vi "Emergency_Stop_JT.vi"(8 "error in":errorcluster, 11 "connection ID":refnum<k5>) -> ()   [LabVIEW 2018]
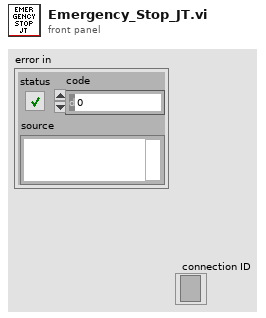
[diagram p1: front panel]
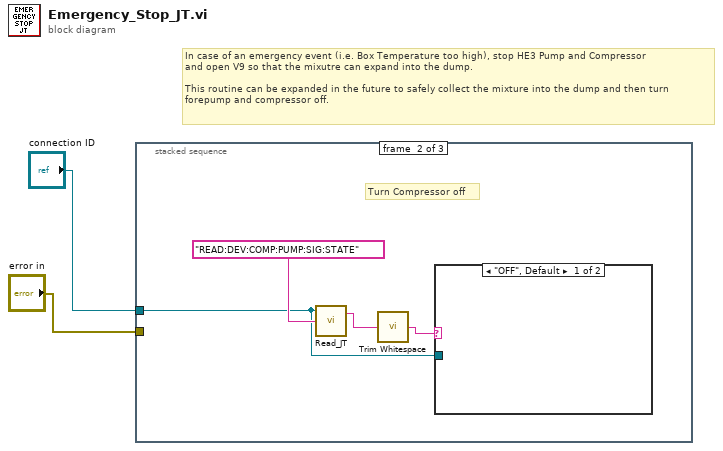
[diagram p0: block diagram]
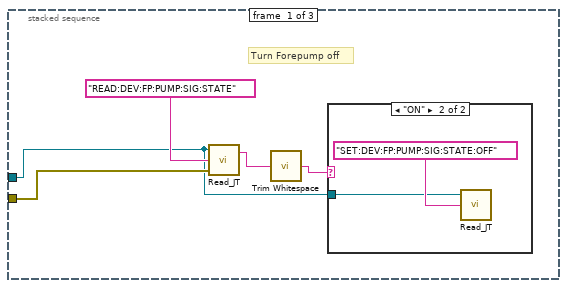
[diagram p2: hidden frame]
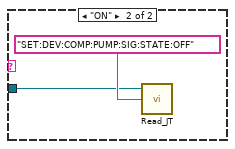
[diagram p4: hidden frame]
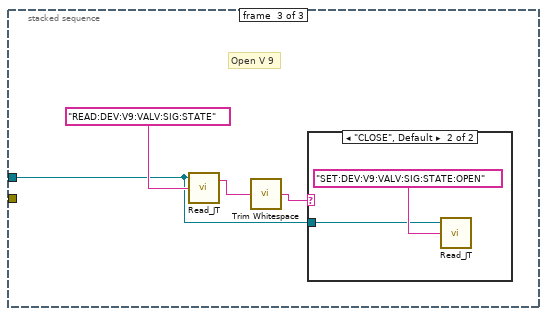
[diagram p5: hidden frame]
diagram:
  # "In case of an emergency event (i.e. Box Temperature too high), stop HE3 Pump and Compressor\nand open V9 so that the mixutre can expand into the dump.\n\nThis routine can be expanded in the future to safely collect the mixture into the dump and then turn \nforepump and compressor off."
  n1 = stacked-sequence {
    tunnel: "connection ID" -> [w3 w12 w18]
    tunnel: "error in" -> [w4 _ _]
    frame #0 {
      # "Turn Forepump off"
      n2 = call "Read_JT.vi"("error in"=w4, "Write"="READ:DEV:FP:PUMP:SIG:STATE", "connection ID"=w3) -> ("Read"=w6:string)  [unwired: 1 in]
      n3 = call <vilib>:"Trim Whitespace.vi"("string"=w6) -> ("trimmed string"=w5:string)  [unwired: 1 in]
      n4 = case shown="\"ON\"" w5 {
        tunnel: w3 -> [_ w8]
        frame "OFF", Default {
        }
        frame "ON" {
          n5 = call "Read_JT.vi"("Write"="SET:DEV:FP:PUMP:SIG:STATE:OFF", "connection ID"=w8) -> ()  [unwired: 2 in, 1 out]
        }
      }
    }
    frame #1 {
      # "Turn Compressor off"
      n6 = call "Read_JT.vi"("Write"="READ:DEV:COMP:PUMP:SIG:STATE", "connection ID"=w12) -> ("Read"=w11:string)  [unwired: 2 in]
      n7 = call <vilib>:"Trim Whitespace.vi"("string"=w11) -> ("trimmed string"=w10:string)  [unwired: 1 in]
      n8 = case shown="\"OFF\", Default" w10 {
        tunnel: w12 -> [_ w14]
        frame "OFF", Default {
        }
        frame "ON" {
          n9 = call "Read_JT.vi"("Write"="SET:DEV:COMP:PUMP:SIG:STATE:OFF", "connection ID"=w14) -> ()  [unwired: 2 in, 1 out]
        }
      }
    }
    frame #2 {
      # "Open V 9"
      n10 = call "Read_JT.vi"("Write"="READ:DEV:V9:VALV:SIG:STATE", "connection ID"=w18) -> ("Read"=w17:string)  [unwired: 2 in]
      n11 = call <vilib>:"Trim Whitespace.vi"("string"=w17) -> ("trimmed string"=w16:string)  [unwired: 1 in]
      n12 = case shown="\"CLOSE\", Default" w16 {
        tunnel: w18 -> [_ w20]
        frame "OPEN" {
        }
        frame "CLOSE", Default {
          n13 = call "Read_JT.vi"("Write"="SET:DEV:V9:VALV:SIG:STATE:OPEN", "connection ID"=w20) -> ()  [unwired: 2 in, 1 out]
        }
      }
    }
  }
